vi "A33ConfigureAM_py.vi"(8 "error in (no error)":errorcluster, 10 "Instrument":string="AG33600A_Gen1", 11 "socket in":refnum<class "zmq_socket.lvclass">) -> (0 "error out":errorcluster, 1 "Standalone":bool, 2 "resulting string":string, 3 "socket out":refnum<class "zmq_socket.lvclass">)   [LabVIEW 2022 SP3]
doc: "Selects the waveform shape, frequency, amplitude, offset, and phase for a standard waveform."
uses:
  <vilib>/addons/zeromq/zmq_socket.lvclass
panel:
  in  "Channel (1: Channel1)":i32(ring)=1 items=["Channel1"=1, "Channel2"=2]
  in  "AM Source (0: Internal)":i32(ring) items=["Internal", "External", "Channel 1", "Channel 2"]
  in  "Modulation Waveform (0: Sine)":i32(ring) items=["Sine", "Square", "Triangle", "Ramp", "Negative Ramp", "Noise", "PRBS", "ARB"]
  in  "Enable Carrier Suppression (F: Disable)":bool
  in  "Enable Amplitude Modulation (T:Enable)":bool=TRUE
  in  "Modulation Depth (100.0 %)":dbl=100.0 format="%#_12g"
  in  "Modulation Frequency (1000.0 Hz)":dbl=1000.0 format="%#_12g"
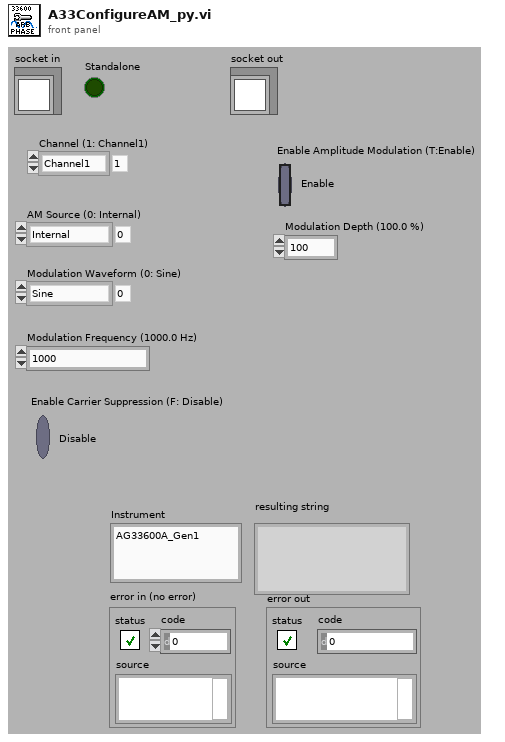
[diagram p1: front panel]
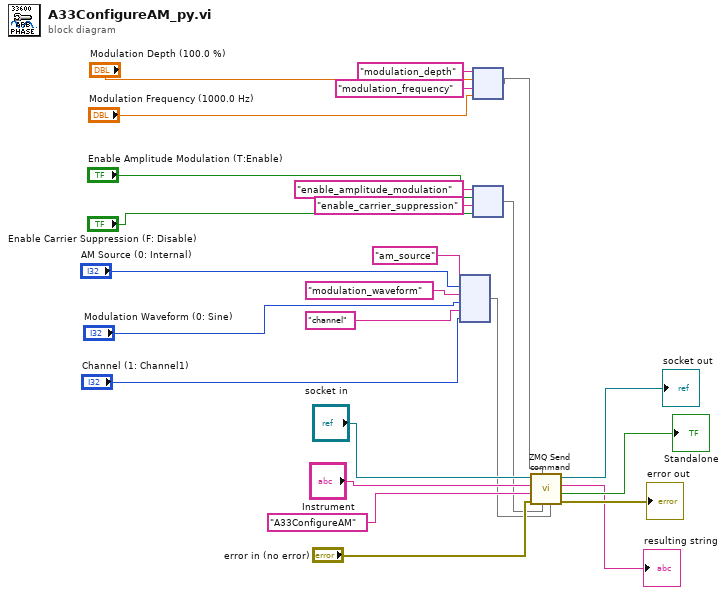
[diagram p0: block diagram]
diagram:
  n1 = node("am_source" ("key"), "AM Source (0: Internal)", "modulation_waveform" ("key"), "Modulation Waveform (0: Sine)", "channel" ("key"), "Channel (1: Channel1)") -> (w1:map{string, i32})
  n2 = node("modulation_depth" ("key"), "Modulation Depth (100.0 %)", "modulation_frequency" ("key"), "Modulation Frequency (1000.0 Hz)") -> (w17:map{string, dbl})
  n3 = node("enable_amplitude_modulation" ("key"), "Enable Amplitude Modulation (T:Enable)", "enable_carrier_suppression" ("key"), "Enable Carrier Suppression (F: Disable)") -> (w8:map{string, bool})
  n4 = call "ZMQ Send command.vi"("Int args"=w1, "Bool args"=w8, "DBL args"=w17, "error in"="error in (no error)", "Command"="A33ConfigureAM", "Instrument"="Instrument", "socket in"="socket in") -> ("error out"=→"error out":errorcluster, "Standalone"=→"Standalone":bool, "Recieved message"=→"resulting string":string, "socket out"=→"socket out":refnum<class "zmq_socket.lvclass">)  [unwired: 1 in]
